vi "Find SLSC Switch Custom Device by Name.vi"(8 "error in":errorcluster, 10 "name":string, 11 "slsc chassis in":T1 format="%.0x") -> (0 "error out":errorcluster, 2 "slsc switch custom device":T1 format="%.0x", 3 "slsc chassis out":T1 format="%.0x")   [LabVIEW 2017, in "NI-SWITCH Scripting.lvlib"]
doc: "Returns the SLSC Switch custom device under the SLSC chassis with the specified name."
uses:
  NI-SWITCH Scripting.lvlib
  Shared/VeriStand SLSC Scripting/VeriStand SLSC Scripting.lvlib
  Shared/Constants.vi
  Shared/NI-SWITCH Shared.lvlib
  <vilib>/NI Veristand/Custom Device API/Custom Device Item Ref.ctl
  <vilib>/NI VeriStand/Custom Device API/Custom Device API.lvlib
panel:
  in  "error message 2":string="The item at the specified slot number is not an SLSC Switch custom device."
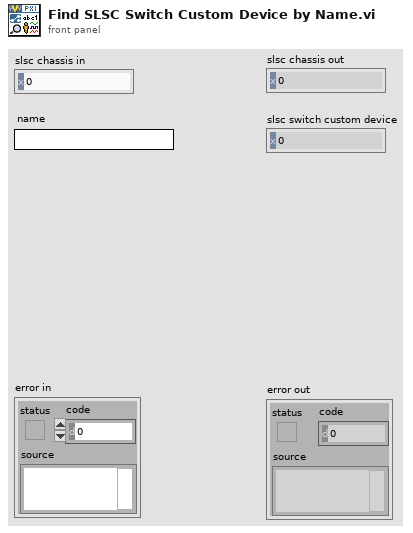
[diagram p1: front panel]
types:
  T1 = typedef "Custom Device API.lvlib/Custom Device Item Ref.ctl" = u64
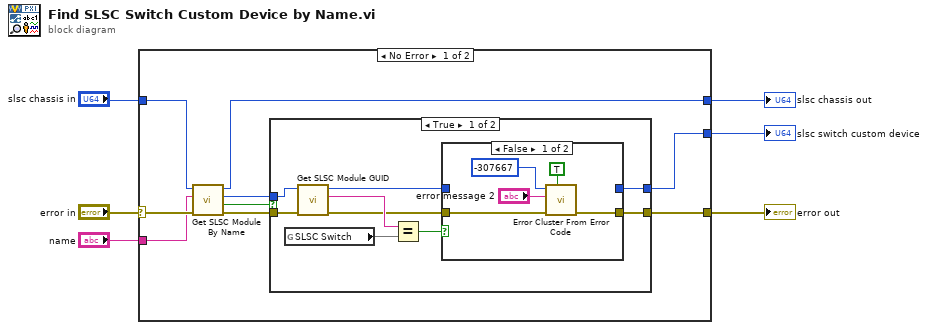
[diagram p0: block diagram]
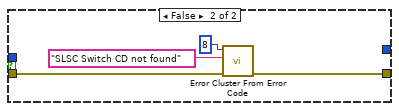
[diagram p3: hidden frame]
diagram:
  n1 = case shown="No Error" "error in" {
    selector: "error in" -> [w15 w37]
    tunnel: [w12 w37] -> w6
    tunnel: "name" -> [w11 _]
    tunnel: [w7 _] -> w3
    tunnel: "slsc chassis in" -> [w10 w36]
    tunnel: [w9 w36] -> w1
    frame No Error {
      n2 = call "Get SLSC Module By Name.vi"("error in (no error)"=w15, "Name"=w11, "SLSC Chassis"=w10) -> ("error out"=w14:errorcluster, "Found"=w13:bool, "SLSC Module"=w8:u64, "SLSC Chassis out"=w9:u64)  [unwired: 5 in]
      n3 = case shown="True" w13 {
        tunnel: [w16 w33] -> w12
        tunnel: w14 -> [w24 w32]
        tunnel: w8 -> [w23 _]
        tunnel: [w17 _] -> w7
        frame True {
          n4 = global read "Constants.vi" "SLSC Switch"() -> (w21)
          n5 = call "Get SLSC Module GUID.vi"("error in (no error)"=w24, "SLSC Module"=w23) -> ("error out"=w20:errorcluster, "Module GUID"=w22:string, "SLSC Module out"=w19:u64)  [unwired: 7 in]
          n6 = Equal?(x=w22, y=w21) -> (x = y?=w18:bool)
          n7 = case shown="False" w18 {
            tunnel: w20 -> [w26 w30]
            tunnel: w19 -> [_ w31]
            tunnel: [_ w31] -> w17
            tunnel: [w25 w30] -> w16
            frame False {
              n8 = call <vilib>:"Error Cluster From Error Code.vi"("show call chain? (False)"=TRUE, "error in (no error)"=w26, "error message (\"\")"="error message 2", "error code (0)"=-307667) -> ("error out"=w25:errorcluster)  [unwired: 5 in]
            }
            frame True {
            }
          }
        }
        frame False {
          n9 = call <vilib>:"Error Cluster From Error Code.vi"("error in (no error)"=w32, "error message (\"\")"="SLSC Switch CD not found" ("error message (\"\")"), "error code (0)"=8) -> ("error out"=w33:errorcluster)  [unwired: 6 in]
        }
      }
    }
    frame Error {
    }
  }
  "error out" <- w6
  "slsc switch custom device" <- w3
  "slsc chassis out" <- w1
